vi "Formula_Node_Ejercicio.vi"() -> ()   [LabVIEW 2020]
panel:
  out "XY Graph":cluster{dbl[], dbl[]}(graph)
  out "Waveform Chart":dbl[](graph)
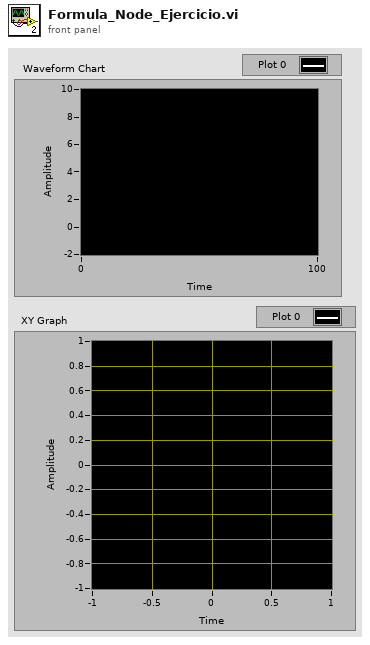
[diagram p1: front panel]
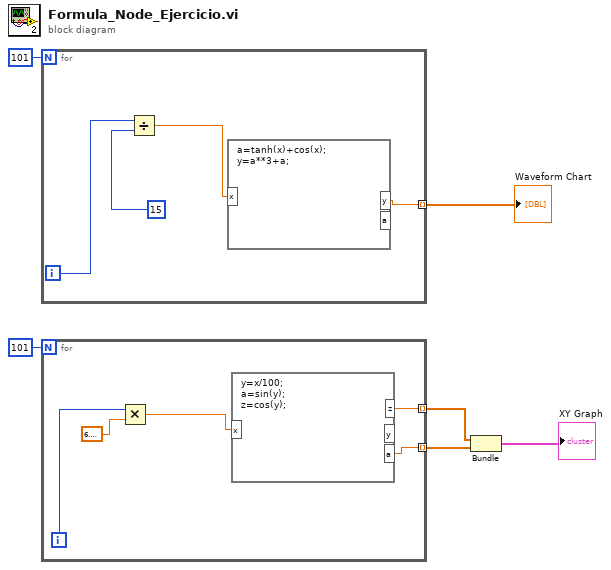
[diagram p0: block diagram]
diagram:
  n1 = for {
    N: 101 -> [_]
    tunnel: [w7] -> w5 mode=indexing
    i -> [w10]
    n2 = Divide(x=w10, y=15) -> (x/y=w8:dbl)
    n3 = formula code="a=tanh(x)+cos(x);\ny=a**3+a;"("x"=w8) -> ("y"=w7:dbl)  [unwired: 1 out]
  }
  "Waveform Chart" <- w5
  n4 = for {
    N: 101 -> [_]
    tunnel: [w12] -> w3 mode=indexing
    tunnel: [w11] -> w2 mode=indexing
    i -> [w15]
    n5 = Multiply(x=w15, y=6.283185307179586) -> (x*y=w13:dbl)
    n6 = formula code="y=x/100;\na=sin(y);\nz=cos(y);"("x"=w13) -> ("a"=w12:dbl, "z"=w11:dbl)  [unwired: 1 out]
  }
  n7 = Bundle(w2, w3) -> (→"XY Graph":cluster{dbl[], dbl[]})  [unwired: 1 in]
